vi "LV2009plus_PostInstall.vi"(8 "error in":errorcluster, 11 "installed files":path[](array[path])) -> (0 "error out":errorcluster)   [LabVIEW 2009]
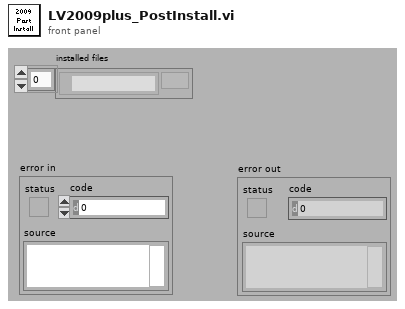
[diagram p1: front panel]
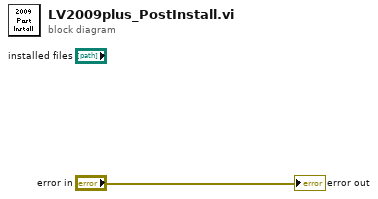
[diagram p0: block diagram]
diagram:
  "error out" <- "error in"
